vi "bus_monitor_server_api.SendStop.vi"(8 "error in (no error)":errorcluster, 11 "gRPC Container in":refnum<class "bus_monitor_server_api.lvclass">) -> (0 "error out":errorcluster, 3 "gRPC Container out":refnum<class "bus_monitor_server_api.lvclass">)   [LabVIEW 2025, in "bus_monitor_server_api.lvlib" / "bus_monitor_server_api.lvclass"]
uses:
  bus_monitor_server_api.lvclass
  bus_monitor_server_api.lvclass/bus_monitor_server_api.ctl
  <vilib>/gRPC/LabVIEW gRPC Servicer/ServiceBase/ServiceBase.lvclass
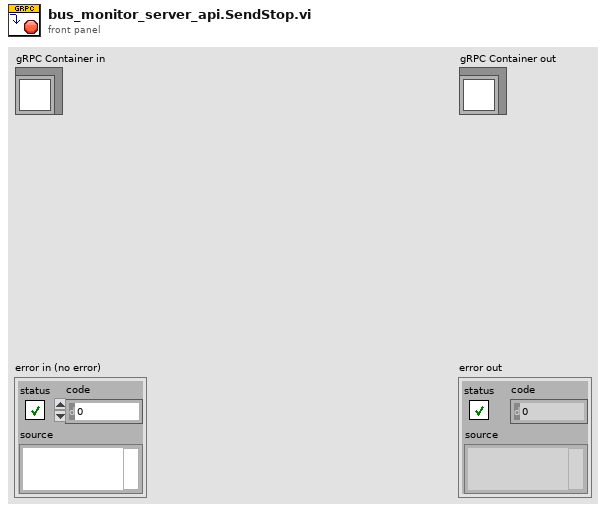
[diagram p1: front panel]
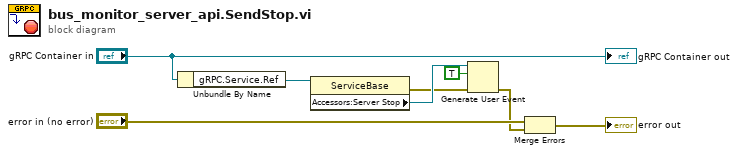
[diagram p0: block diagram]
diagram:
  n1 = Unbundle By Name("gRPC Container in") -> ("gRPC.Service.Ref"=w3:refnum<class "ServiceBase.lvclass">)
  n2 = property class="ServiceBase"(reference=w3) -> (error out=w1:errorcluster, "Accessors:Server Stop"=w2:refnum<user-event>)  [unwired: 1 in, 1 out]
  n3 = Generate User Event(user event=w2, event data cluster=TRUE ("notification"), error in=w1) -> (error out=w4:errorcluster)  [unwired: 1 in, 1 out]
  n4 = Merge Errors("error in (no error)", w4) -> (→"error out":errorcluster)
  "gRPC Container out" <- "gRPC Container in"
